vi "DRAW_Mouse_DAQmx_w_overlay.vi"(1 "Overlay track show state":u32, 4 "Reset buffers? (F)":bool, 5 "Overlays cluster":T1, 6 "Error In (no error)":errorcluster, 7 "Mouse position":T4, 8 "Size of the image (480x480)":T5={"Numeric Control"=480.0, "Numeric Control"=480.0}, 9 "Mouse drawing parameters":T2, 10 "Image In":T3) -> (0 "Error Out":errorcluster, 2 "Reset buffers out":bool, 3 "Image Out":T3)   [LabVIEW 2018, in "Tracker.lvlib"]
uses:
  Tracker.lvlib
  Controls/CTL_Animal_Coordinates_and_Speed.ctl
  <vilib>/vision/Image Controls.llb/IMAQ Image.ctl
  Controls/CTL_Mouse_Draw_Params.ctl
  Controls/CTL_Overlays_cluster.ctl
  <vilib>/Utility/miscctls.llb/LVBoundsTypeDef.ctl
  69540c99-c38e-483f-99b2-6b34fe281cd1.vi
  0fd21f04-c3bc-483a-b466-79e3f59440e3.vi
  69540c99-c38e-483f-99b2-6b34fe281cd1.vi/177b33a1-ea6e-4d83-abe8-c6c728c9b885.vi
panel:
  in  "Experiment Diagram":T3(plugin-control)=refnum
  out "Colors array input":u32[](array[colorbox])
  out "Rainbow colors":bool=TRUE
  in  "Trace color 2":u32(colorbox)
  in  "Trace color":u32(colorbox)=16757314
  out "Bright mouse lineout":bool=TRUE
  in  "Mouse lineout color":u32(colorbox)=16775210
  in  "Iris size factor":dbl=0.05000000000000001 min=0.01 max=0.22 step=0.005 format="%#_13g"
  in  "Eye size factor":dbl=0.07000000000000002 min=0.02 max=0.24 step=0.01 format="%#_13g"
  out "Mouse abs. coordinates, pix":T5={"Numeric Control"=240.0, "Numeric Control"=240.0}
  in  "Mouse color":u32(colorbox)=5460819
  in  "Mouse length, mm":dbl=40.0
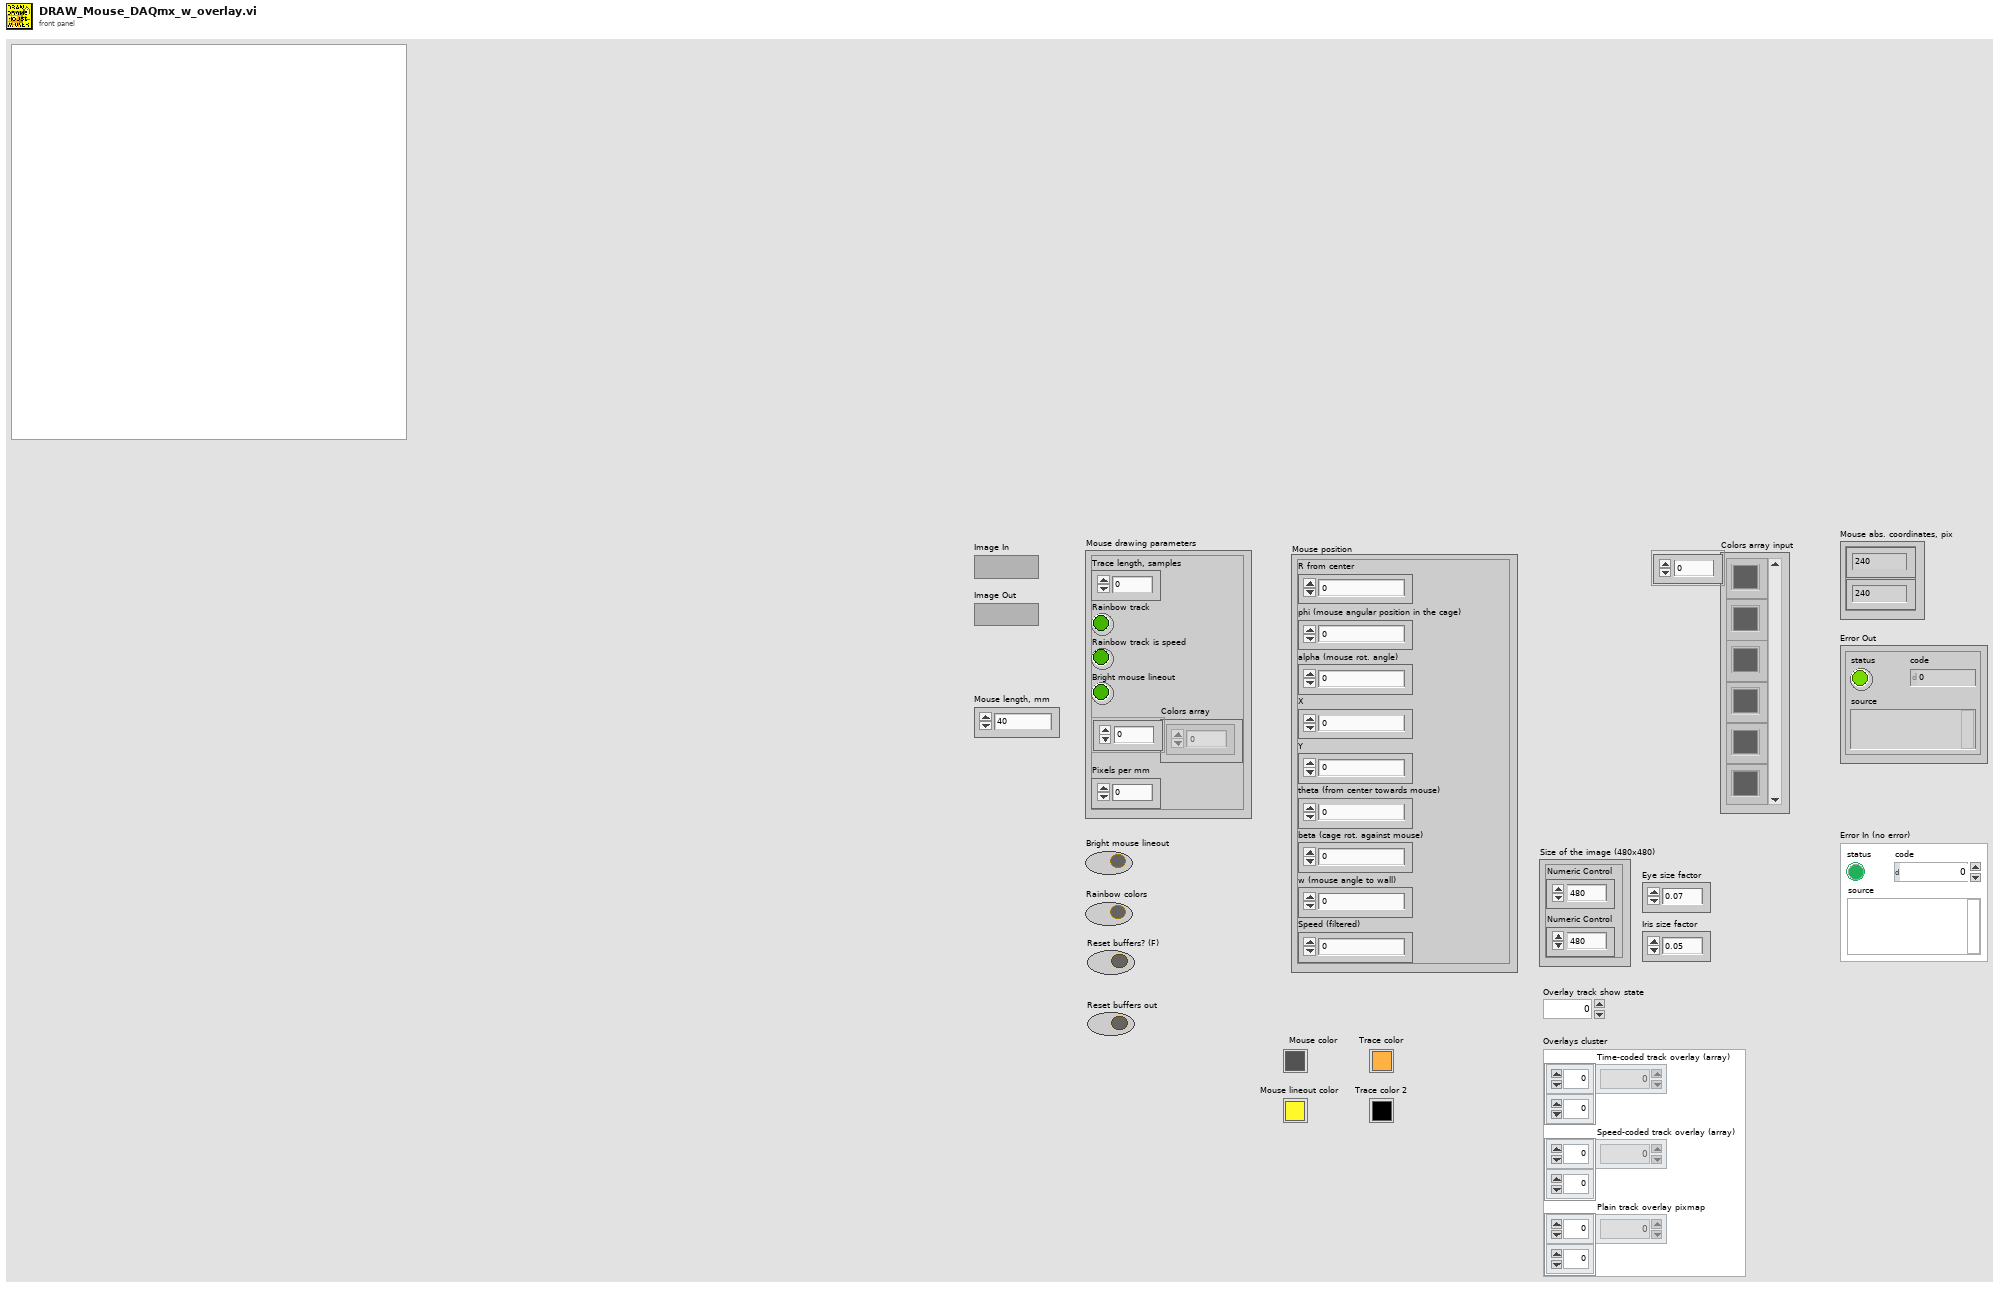
[diagram p1: front panel]
types:
  T1 = typedef "Tracker.lvlib/CTL_Overlays_cluster.ctl" = cluster{"Time-coded track overlay (array)":u32[][], "Speed-coded track overlay (array)":u32[][], "Plain track overlay pixmap":u32[][]}
  T2 = typedef "Tracker.lvlib/CTL_Mouse_Draw_Params.ctl" = cluster{"Trace length, samples":u16, "Rainbow track":bool, "Rainbow track is speed":bool, "Bright mouse lineout":bool, "Colors array":u32[], "Pixels per mm":dbl}
  T3 = typedef "IMAQ Image.ctl" = refnum<image>
  T4 = typedef "Tracker.lvlib/CTL_Animal_Coordinates_and_Speed.ctl" = cluster{"R from center":dbl, "phi (mouse angular position in the cage)":dbl, "alpha (mouse rot. angle)":dbl, "X":dbl, "Y":dbl, "theta (from center towards mouse)":dbl, "beta (cage rot. against mouse)":dbl, "w (mouse angle to wall)":dbl, "Speed (filtered)":dbl}
  T5 = cluster{"Numeric Control":dbl, "Numeric Control":dbl}
  T6 = typedef "LVBoundsTypeDef.ctl" = cluster{"Width":u32, "Height":u32}
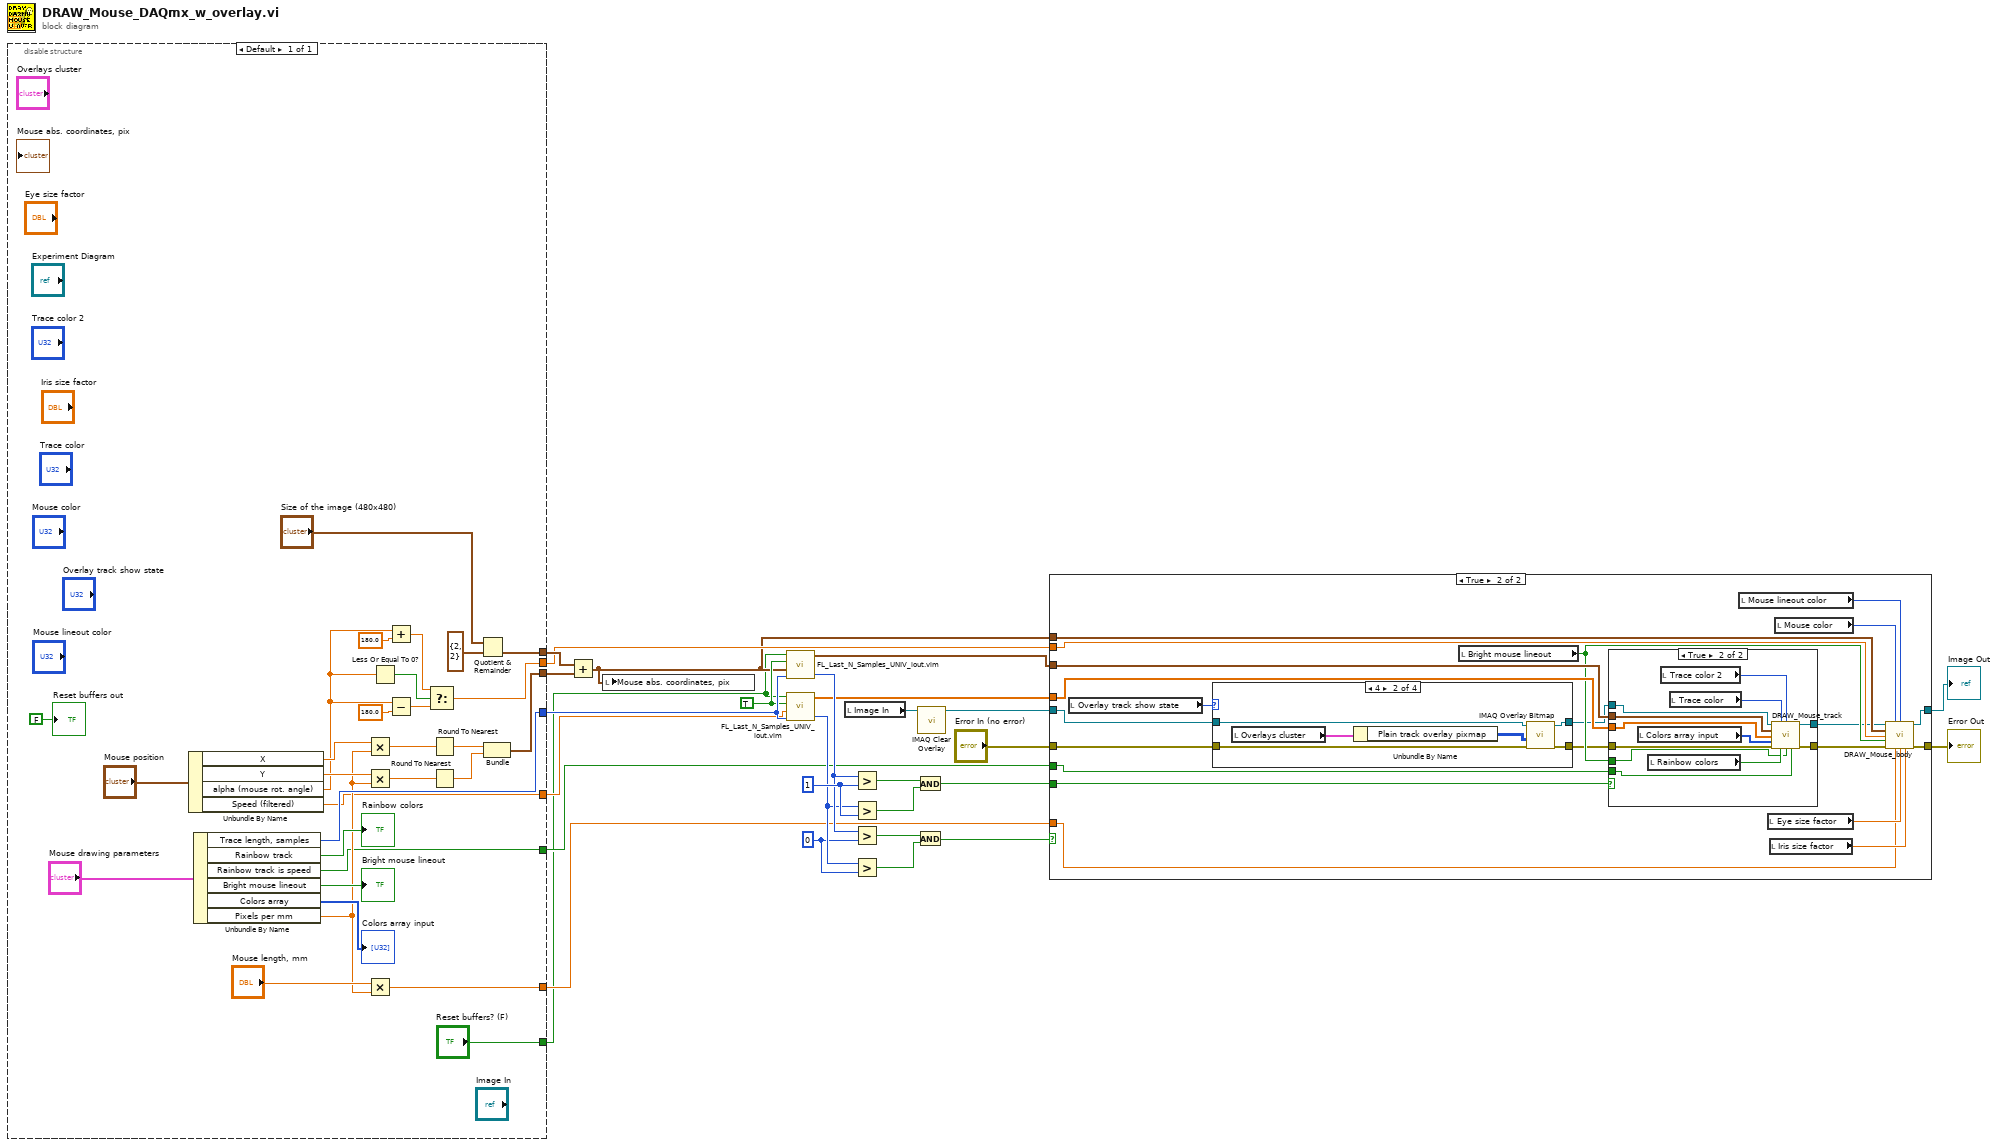
[diagram p0: block diagram]
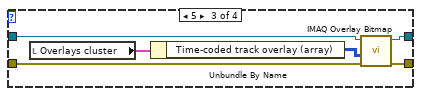
[diagram p4: hidden frame]
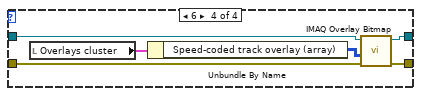
[diagram p5: hidden frame]
diagram:
  w17 = 0 ("y")
  w21 = 1 ("y")
  w25 = TRUE ("Flip buffer output (F)")
  n1 = disable-structure shown="Default" {
    disable-tunnel: [w46] -> w10
    disable-tunnel: [w52] -> w27
    disable-tunnel: [w40] -> w26
    disable-tunnel: [w35] -> w24
    disable-tunnel: [w34] -> w4
    disable-tunnel: [w31] -> w20
    disable-tunnel: [w30] -> w11
    disable-tunnel: ["Reset buffers? (F)"] -> w1
    frame Enabled {
      n2 = Unbundle By Name("Mouse position") -> ("X"=w44:dbl, "Y"=w43:dbl, "alpha (mouse rot. angle)"=w42:dbl, "Speed (filtered)"=w35:dbl)
      n3 = Unbundle By Name("Mouse drawing parameters") -> ("Trace length, samples"=w40:u16, "Rainbow track"=→"Rainbow colors":bool, "Rainbow track is speed"=w34:bool, "Bright mouse lineout"=→"Bright mouse lineout":bool, "Colors array"=→"Colors array input":u32[], "Pixels per mm"=w36:dbl)
      n4 = Multiply(x=w44, y=w36) -> (x*y=w56:dbl)
      n5 = Multiply(x=w43, y=w36) -> (x*y=w55:dbl)
      n6 = Multiply(x="Mouse length, mm", y=w36) -> (x*y=w30:dbl)
      n7 = Less Or Equal To 0?(x=w42) -> (x <= 0?=w51:bool)
      n8 = Add(x=w42, y=sgl 180.0) -> (x+y=w48:dbl)
      n9 = Subtract(x=w42, y=sgl 180.0) -> (x-y=w50:dbl)
      n10 = Select(t=w48, s=w51, f=w50) -> (s? t:f=w46:dbl)
      n11 = Round To Nearest(number=w56) -> (nearest integer value=w54:dbl)
      n12 = Round To Nearest(number=w55) -> (nearest integer value=w53:dbl)
      n13 = Quotient & Remainder(x="Size of the image (480x480)", y=T6 {"Width"=2, "Height"=2}) -> (floor(x/y)=w31:cluster{dbl, dbl})  [unwired: 1 out]
      n14 = Bundle(w54, w53) -> (w52:cluster{dbl, dbl})  [unwired: 1 in]
      "Reset buffers out" <- FALSE ("Reset buffers out")
    }
  }
  n15 = Add(x=w20, y=w27) -> (x+y=w9:cluster{dbl, dbl})
  n16 = local write "Mouse abs. coordinates, pix"(w9) -> ()
  n17 = call "FL_Last_N_Samples_UNIV_iout.vim"("Buffer length, samples"=w26, "Input sample"=w9, "Flip buffer output (F)"=w25, "Reset buffer"=w1) -> ("Current buffer length, samples"=w19:i32, "Output Array"=w6:cluster{"X":dbl, "Y":dbl}[])  [unwired: 1 out]
  n18 = call "FL_Last_N_Samples_UNIV_iout.vim"("Buffer length, samples"=w26, "Input sample"=w24, "Flip buffer output (F)"=w25, "Reset buffer"=w1) -> ("Current buffer length, samples"=w18:i32, "Output Array"=w5:dbl[])  [unwired: 1 out]
  n19 = local read "Image In"() -> (w13:T3)
  n20 = Greater?(x=w19, y=w21) -> (0:w23:bool)
  n21 = Greater?(x=w18, y=w21) -> (0:w22:bool)
  n22 = Greater?(x=w19, y=w17) -> (0:w16:bool)
  n23 = Greater?(x=w18, y=w17) -> (0:w15:bool)
  n24 = And(x=w23, y=w22) -> (x .and. y?=w8:bool)
  n25 = And(x=w16, y=w15) -> (x .and. y?=w14:bool)
  n26 = call "IMAQ Clear Overlay"("Image"=w13) -> ("Image Out"=w12:T3)  [unwired: 9 in, 1 out]
  n27 = case shown="True" w14 {
    tunnel: w12 -> [w59 w68]
    tunnel: w11 -> [_ w76]
    tunnel: w10 -> [_ w75]
    tunnel: w9 -> [_ w73]
    tunnel: w8 -> [_ w74]
    tunnel: [w59 w60] -> w7
    tunnel: w6 -> [_ w72]
    tunnel: w5 -> [_ w71]
    tunnel: w4 -> [_ w69]
    tunnel: [w58 w61] -> w3
    tunnel: "Error In (no error)" -> [w58 w66]
    frame False {
    }
    frame True {
      n28 = local read "Overlay track show state"() -> (w67:u32)
      n29 = case shown="4" w67 {
        tunnel: w68 -> [w82 w88 w94 w100]
        tunnel: [w82 w87 w93 w99] -> w65
        tunnel: w66 -> [w81 w84 w90 w96]
        tunnel: [w81 w83 w89 w95] -> w64
        frame 0..3, 7, Default {
        }
        frame 4 {
          n30 = local read "Overlays cluster"() -> (w86:T1)
          n31 = Unbundle By Name(w86) -> ("Plain track overlay pixmap"=w85:u32[][])
          n32 = call "IMAQ Overlay Bitmap"("error in (no error)"=w84, "Bitmap"=w85, "Image"=w88) -> ("error out"=w83:errorcluster, "Image Out"=w87:T3)  [unwired: 7 in]
        }
        frame 5 {
          n33 = local read "Overlays cluster"() -> (w92:T1)
          n34 = Unbundle By Name(w92) -> ("Time-coded track overlay (array)"=w91:u32[][])
          n35 = call "IMAQ Overlay Bitmap"("error in (no error)"=w90, "Bitmap"=w91, "Image"=w94) -> ("error out"=w89:errorcluster, "Image Out"=w93:T3)  [unwired: 7 in]
        }
        frame 6 {
          n36 = local read "Overlays cluster"() -> (w98:T1)
          n37 = Unbundle By Name(w98) -> ("Speed-coded track overlay (array)"=w97:u32[][])
          n38 = call "IMAQ Overlay Bitmap"("error in (no error)"=w96, "Bitmap"=w97, "Image"=w100) -> ("error out"=w95:errorcluster, "Image Out"=w99:T3)  [unwired: 7 in]
        }
      }
      n39 = local read "Bright mouse lineout"() -> (w70:bool)
      n40 = case shown="True" w74 {
        tunnel: w65 -> [w102 w112]
        tunnel: [w102 w111] -> w63
        tunnel: w72 -> [_ w110]
        tunnel: w71 -> [_ w109]
        tunnel: w70 -> [_ w106]
        tunnel: w69 -> [_ w105]
        tunnel: w64 -> [w101 w104]
        tunnel: [w101 w103] -> w62
        frame False {
        }
        frame True {
          n41 = local read "Colors array input"() -> (w108:u32[])
          n42 = local read "Rainbow colors"() -> (w107:bool)
          n43 = local read "Trace color 2"() -> (w114:u32)
          n44 = local read "Trace color"() -> (w113:u32)
          n45 = call "DRAW_Mouse_track.vi"("Image ref. in"=w112, "Trace color"=w113, "Trace color 2"=w114, "Track array in"=w110, "Speed array in"=w109, "Colors array input"=w108, "Error In (no error)"=w104, "Rainbow colors"=w107, "Bright mouse lineout"=w106, "Rainbow track is speed"=w105) -> ("Image ref. out"=w111:T3, "Error Out"=w103:errorcluster)  [unwired: 4 in]
        }
      }
      n46 = local read "Mouse lineout color"() -> (w80:u32)
      n47 = local read "Eye size factor"() -> (w77:dbl)
      n48 = local read "Iris size factor"() -> (w78:dbl)
      n49 = local read "Mouse color"() -> (w79:u32)
      n50 = call "DRAW_Mouse_body.vi"("Refnum in"=w63, "Mouse color"=w79, "Mouse lineout color"=w80, "Mouse position, pix"=w73, "Mouse rotation angle, deg"=w75, "Bright mouse lineout"=w70, "Error In (no error)"=w62, "Mouse size, pix"=w76, "Eye size factor"=w77, "Iris size factor"=w78) -> ("Image ref. out"=w60:T3, "Error Out"=w61:errorcluster)  [unwired: 4 in]
    }
  }
  "Image Out" <- w7
  "Error Out" <- w3
